vi "ListAllFolderIterate.vi"(11 "Path":path) -> (3 "PathArray":path[](array[path]))   [LabVIEW 2014]
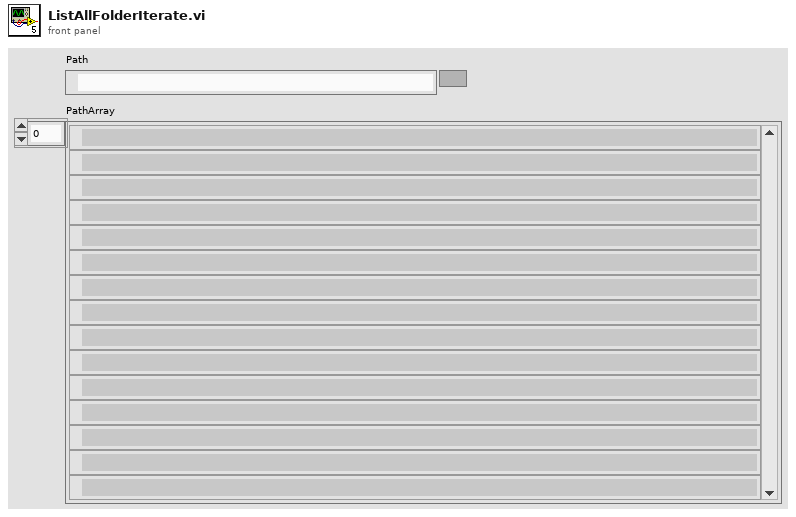
[diagram p1: front panel]
types:
  T1 = cluster{"StackArray":cluster{"path out":path, "folder names":string[]}[], "CurrentPath":path, "FolderArray":string[], "Result":path[]}
  T2 = cluster{"path out":path, "folder names":string[]}[]
  T3 = cluster{"CurrentPath":path, "FolderArray":string[]}
  T4 = cluster{"path out":path, "folder names":string[]}
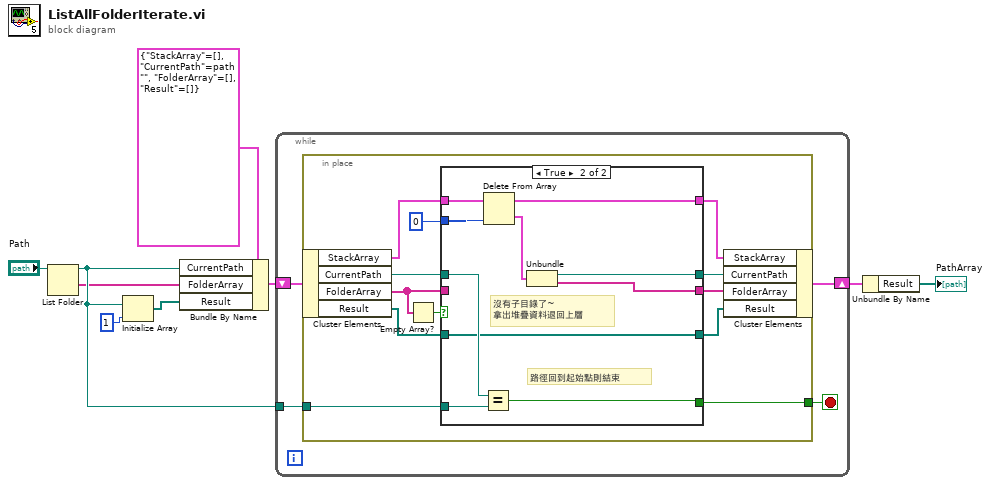
[diagram p0: block diagram]
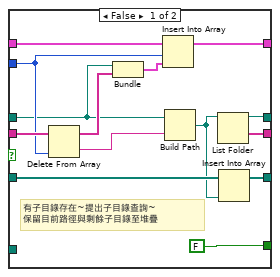
[diagram p2: hidden frame]
diagram:
  n1 = List Folder(path="Path") -> (path out=w5:path, folder names=w4:string[])  [unwired: 3 in, 2 out]
  n2 = Initialize Array(w5, 1 ("dimension size")) -> (w3:path[])
  n3 = Bundle By Name(cluster=T1 {"StackArray"=[], "CurrentPath"=path "", "FolderArray"=[], "Result"=[]}, "CurrentPath"=w5, "FolderArray"=w4, "Result"=w3) -> (w6:T1)
  n4 = while {
    tunnel: w5 -> [w13]
    shift-right: [w10] -> w2
    shift-left: w6 -> [w11]
    stop <- w12 stop-if-true
    n5 = in-place {
      in-place-border: w13 -> [w25]
      in-place-border: [w23] -> w12
      n6 = in-place-cluster #1(w11) -> ("StackArray"=w18:T2, "CurrentPath"=w19:path, "FolderArray"=w20:string[], "Result"=w21:path[])
      n7 = Empty Array?(array=w20) -> (empty?=w24:bool)
      n8 = case shown="True" w24 {
        tunnel: w19 -> [w29 w42]
        tunnel: w20 -> [w39 _]
        tunnel: [w34 w41] -> w15
        tunnel: [w33 w46] -> w16
        tunnel: [w35 w48] -> w14
        tunnel: w18 -> [w36 w49]
        tunnel: [FALSE w43] -> w23
        tunnel: 0 ("dimension size") -> [w30 w45]
        tunnel: w25 -> [_ w44]
        tunnel: [w27 w40] -> w17
        tunnel: w21 -> [w28 w40]
        frame False {
          # "有子目錄存在~提出子目錄查詢~\n保留目前路徑與剩餘子目錄至堆疊"
          n9 = Delete From Array(array=w39, index=w30) -> (deleted portion=w38:string, array with subset deleted=w37:string[])  [unwired: 1 in]
          n10 = Bundle("CurrentPath"=w29, "FolderArray"=w37) -> (w31:T3)  [unwired: 1 in]
          n11 = Insert Into Array(array=w36, index=w30, new element=w31) -> (w35:T2)
          n12 = Build Path(base path=w29, name or relative path=w38) -> (appended path=w26:path)
          n13 = List Folder(path=w26) -> (path out=w34:path, folder names=w33:string[])  [unwired: 3 in, 2 out]
          n14 = Insert Into Array(array=w28, new element=w26) -> (w27:path[])  [unwired: 1 in]
        }
        frame True {
          # "路徑回到起始點則結束"
          # "沒有子目錄了~\n拿出堆疊資料退回上層"
          n15 = Equal?(x=w42, y=w44) -> (x = y?=w43:bool)
          n16 = Delete From Array(array=w49, index=w45) -> (deleted portion=w47:T4, array with subset deleted=w48:T2)  [unwired: 1 in]
          n17 = Unbundle(w47) -> ("path out"=w41:path, "folder names"=w46:string[])
        }
      }
      n18 = in-place-cluster #1("StackArray"=w14, "CurrentPath"=w15, "FolderArray"=w16, "Result"=w17) -> (w10:T1)
    }
  }
  n19 = Unbundle By Name(w2) -> ("Result"=→"PathArray":path[])
